vi "Highlight Possible Moves.vi"(8 "error in (no error)":errorcluster, 11 "Reversi in":refnum<class "Reversi.lvclass">) -> (0 "error out":errorcluster, 3 "Reversi out":refnum<class "Reversi.lvclass">)   [LabVIEW 2020, in "Reversi.lvlib" / "Reversi.lvclass"]
uses:
  Reversi.lvclass
  Reversi.lvclass/Reversi.ctl
  Space Ring.ctl
panel:
  # "This VI highlights all possible moves if the boolean is toggled."
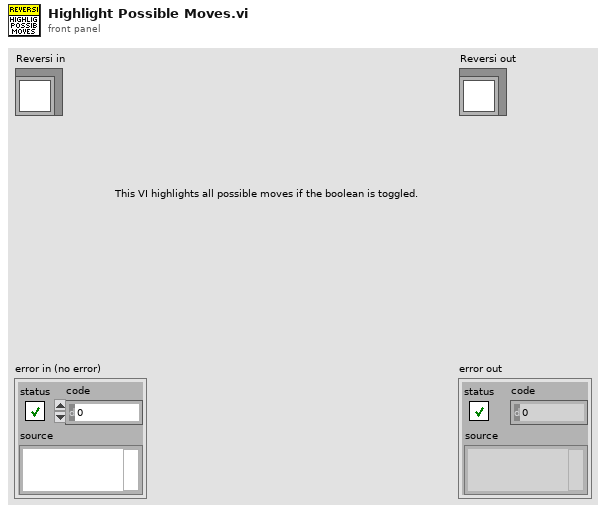
[diagram p1: front panel]
types:
  T1 = typedef "Reversi.lvlib/Reversi.lvclass/Space Ring.ctl" = u16
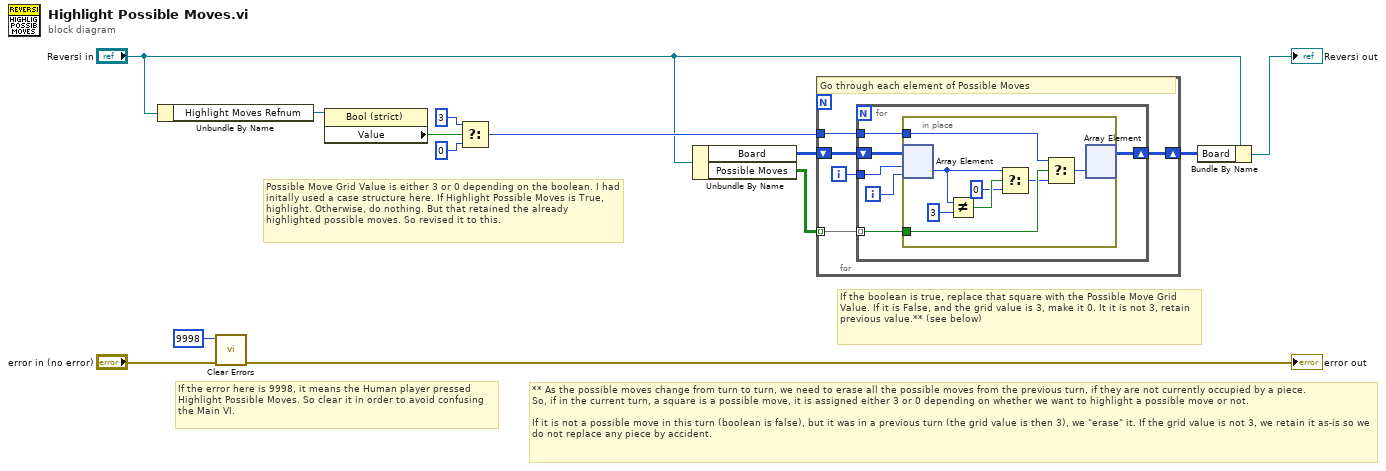
[diagram p0: block diagram]
diagram:
  # "If the boolean is true, replace that square with the Possible Move Grid Value. If it is False, and the grid value is 3, make it 0. It it is not 3, retain previous value.** (see below)"
  # "Possible Move Grid Value is either 3 or 0 depending on the boolean. I had initally used a case structure here. If Highlight Possible Moves is True, highlight. Otherwise, do nothing. But that retained the already highlighted possible moves. So revised it to this."
  # "If the error here is 9998, it means the Human player pressed Highlight Possible Moves. So clear it in order to avoid confusing the Main VI."
  # "** As the possible moves change from turn to turn, we need to erase all the possible moves from the previous turn, if they are not currently occupied by a piece.\nSo, if in the current turn, a square is a possible move, it is assigned either 3 or 0 depending on whether we want to highlight a possible move or not.\n\nIf it is not a possible move in this turn (boolean is false), but it was in a previous turn (the grid value is then 3), we \"erase\" it. If the grid value is not 3, we retain it as-is so we do not replace any piece by accident."
  n1 = Unbundle By Name("Reversi in") -> ("Highlight Moves Refnum"=w11:refnum<vi>)
  n2 = call <vilib>:"Clear Errors.vi"("error in (no error)"="error in (no error)", "specific error code to clear (0: all)"=9998) -> ("error out"=→"error out":errorcluster)  [unwired: 4 in, 1 out]
  n3 = property class="Bool (strict)"(reference=w11) -> ("Value"=w10:bool)  [unwired: 1 in, 2 out]
  n4 = Select(t=T1 3 ("y"), s=w10, f=T1 0) -> (s? t:f=w7:T1)
  n5 = Unbundle By Name("Reversi in") -> ("Board"=w4:T1[][], "Possible Moves"=w2:bool[][])
  n6 = for {
    shift-right: [w17] -> w3
    shift-left: w4 -> [w18]
    tunnel: w2 -> [w16] mode=indexing
    tunnel: w7 -> [w14]
    i -> [w15]
    # "Go through each element of Possible Moves"
    n7 = for {
      shift-right: [w23] -> w17
      shift-left: w18 -> [w24]
      tunnel: w16 -> [w20] mode=indexing
      tunnel: w15 -> [w22]
      tunnel: w14 -> [w19]
      i -> [w21]
      n8 = in-place {
        in-place-border: w20 -> [w31]
        in-place-border: w19 -> [w25]
        # "If the boolean is true, replace that square with the Possible Move Grid Value. If it is False, and the grid value is 3, make it 0. It it is not 3, retain previous value.** (see below)"
        n9 = in-place-array #1(w24, w22, w21) -> (w28:T1)
        n10 = Not Equal?(x=w28, y=T1 3) -> (x != y?=w30:bool)
        n11 = Select(t=w28, s=w30, f=T1 0) -> (s? t:f=w26:T1)
        n12 = Select(t=w25, s=w31, f=w26) -> (s? t:f=w32:T1)
        n13 = in-place-array #1(w32) -> (w23:T1[][])  [unwired: 2 out]
      }
    }
  }
  n14 = Bundle By Name(cluster="Reversi in", "Board"=w3) -> (→"Reversi out":refnum<class "Reversi.lvclass">)
